vi "TestItemTo3Cam.vi"(0 "量测内容":string[][](array[string])) -> (3 "3只相机量测规格(不含取消的测试项目)":T4 {"相机4量测规格"."上限" format="%#.4g"; "相机4量测规格"."下限" format="%#.4g"; "相机3量测规格"."上限" format="%#.4g"; "相机3量测规格"."下限" format="%#.4g"; "相机2量测规格"."上限" format="%#.4g"; "相机2量测规格"."下限" format="%#.4g"; "相机1量测规格"."上限" format="%#.4g"; "相机1量测规格"."下限" format="%#.4g"}, 4 "各相机光源有效量测项目":T1, 6 "4只相机是否拍照":bool[](array[boolean]))   [LabVIEW 2014]
uses:
  CamLight.ctl
  Controls/TestThreshold.ctl
panel:
  out "数组 2":enum32{"相机1", "相机2", "相机3", "相机4"}[](array[ring])
  out "数组":bool[](array[boolean])
  out "第一次拍照组合":T2[](array[typedef])
  # "~"
  # "~"
  # "~"
  # "~"
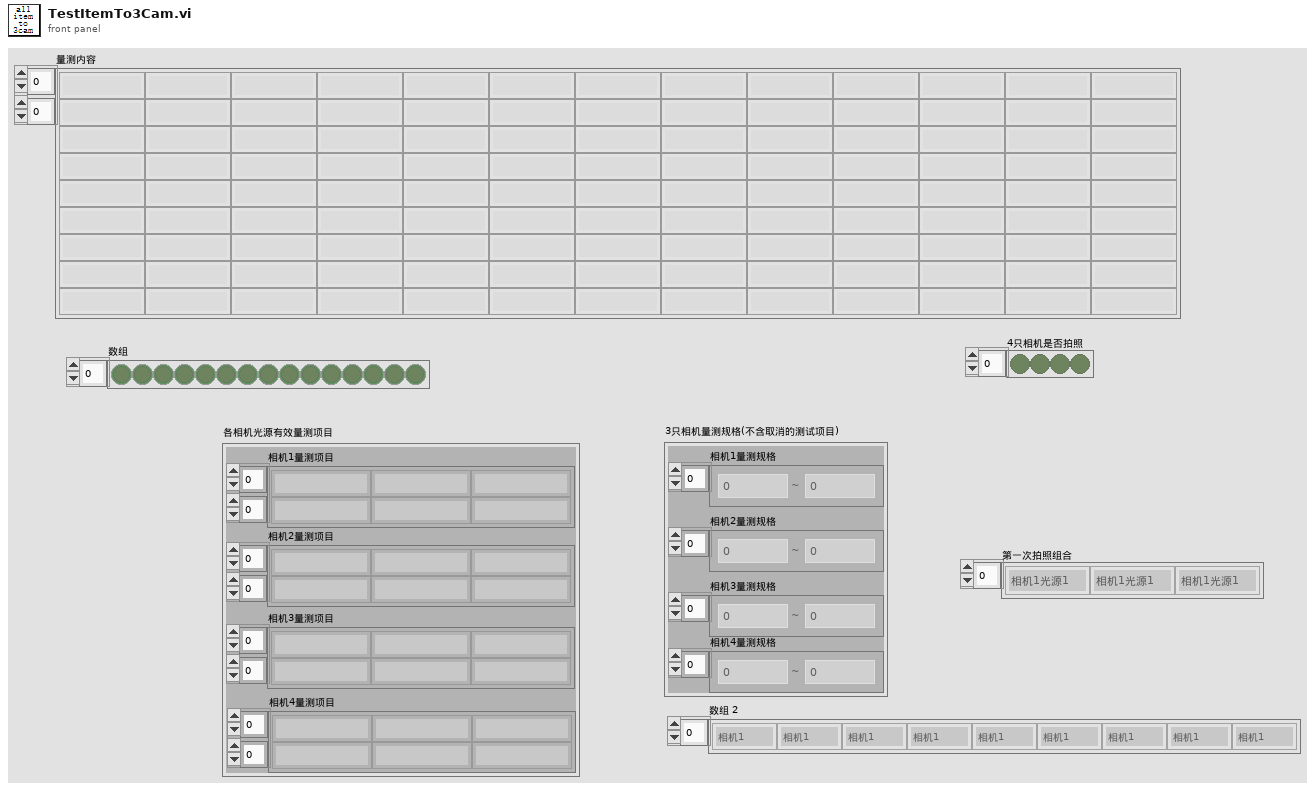
[diagram p1: front panel]
types:
  T1 = cluster{"相机1量测项目":string[][], "相机2量测项目":string[][], "相机3量测项目":string[][], "相机4量测项目":string[][]}
  T2 = typedef "CamLight.ctl" = enum16{"相机1光源1", "相机2光源2", "相机3光源3", "相机4光源4", "None"}
  T3 = typedef "TestThreshold.ctl" = cluster{"下限":dbl, "上限":dbl}
  T4 = cluster{"相机1量测规格":T3[], "相机2量测规格":T3[], "相机3量测规格":T3[], "相机4量测规格":T3[]}
  T5 = typedef "锁附点位信息.ctl" = cluster{"点位名称":string, "点位坐标(图纸)":T6, "点位坐标(实际)":T6, "补偿值":T6, "锁附时机械手角度":T7, "选择螺丝供料机":enum32{"1号供料机", "2号供料机", "3号供料机", "4号供料机"}}
  T6 = typedef "锁附点位坐标XYZ.ctl" = cluster{"X":dbl, "Y":dbl, "Z":dbl}
  T7 = typedef "锁附时机械手角度.ctl" = enum16{"0度", "90度", "180度", "270度"}
  T8 = cluster{string[][], string[][], string[][], string[][]}
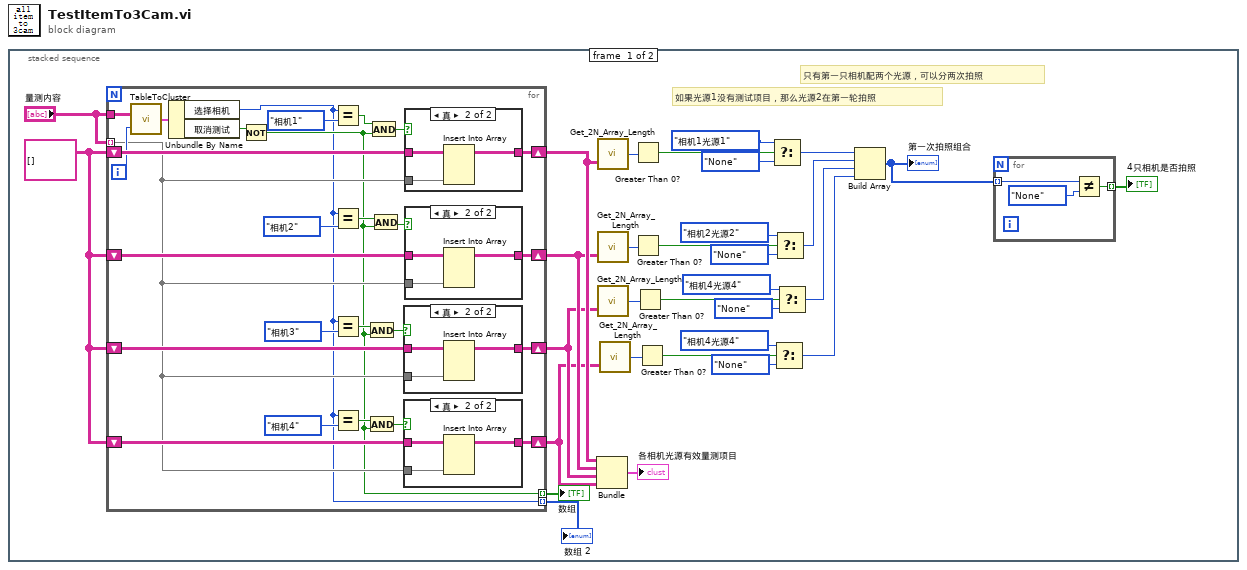
[diagram p0: block diagram]
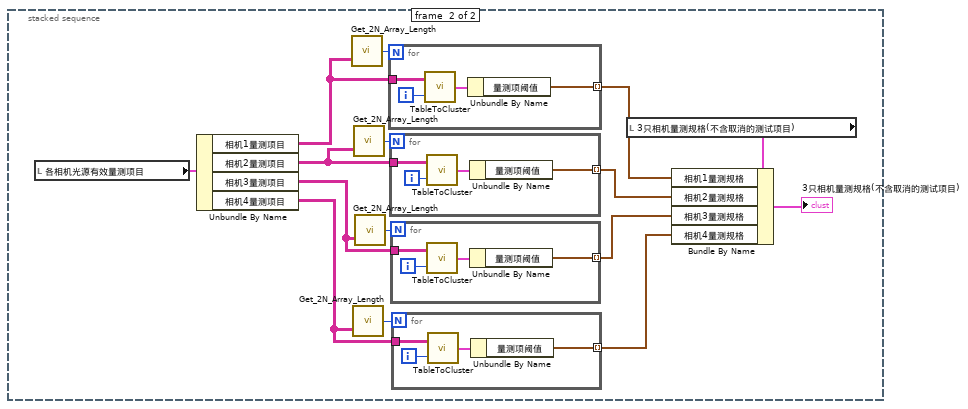
[diagram p6: hidden frame]
diagram:
  n1 = stacked-sequence {
    frame #0 {
      w12 = string[][] []
      # "只有第一只相机配两个光源，可以分两次拍照"
      # "如果光源1没有测试项目，那么光源2在第一轮拍照"
      n2 = for {
        tunnel: "量测内容" -> [w55]
        shift-right: [w60] -> w18
        shift-left: w12 -> [w61]
        shift-right: [w59] -> w17
        shift-left: w12 -> [w58]
        shift-right: [w57] -> w16
        shift-left: w12 -> [w56]
        tunnel: "量测内容" -> [w41] mode=indexing
        shift-right: [w42] -> w10
        shift-left: w12 -> [w43]
        tunnel: [w36] -> w2 mode=indexing
        tunnel: [w35] -> w1 mode=indexing
        i -> [w54]
        n3 = call "TableToCluster.vi"("Row"=w54, "锁附点位信息表"=w55) -> ("锁附点位信息"=w53:T5)
        n4 = Unbundle By Name(w53) -> ("选择相机"=w35:enum32{"相机1", "相机2", "相机3", "相机4"}, "取消测试"=w52:bool)
        n5 = Not(x=w52) -> (.not. x?=w36:bool)
        n6 = Equal?(x=w35, y=enum32{"相机1", "相机2", "相机3", "相机4"}."相机1") -> (x = y?=w51:bool)
        n7 = Equal?(x=w35, y=enum32{"相机1", "相机2", "相机3", "相机4"}."相机2") -> (x = y?=w49:bool)
        n8 = Equal?(x=w35, y=enum32{"相机1", "相机2", "相机3", "相机4"}."相机3") -> (x = y?=w47:bool)
        n9 = Equal?(x=w35, y=enum32{"相机1", "相机2", "相机3", "相机4"}."相机4") -> (x = y?=w44:bool)
        n10 = And(x=w47, y=w36) -> (x .and. y?=w46:bool)
        n11 = And(x=w44, y=w36) -> (x .and. y?=w45:bool)
        n12 = And(x=w51, y=w36) -> (x .and. y?=w50:bool)
        n13 = And(x=w49, y=w36) -> (x .and. y?=w48:bool)
        n14 = case shown="真" w46 {
          tunnel: w41 -> [_ w68]
          tunnel: w56 -> [w66 w69]
          tunnel: [w66 w67] -> w57
          frame False {
          }
          frame True {
            n15 = Insert Into Array(array=w69, new element=w68) -> (w67:string[][])  [unwired: 2 in]
          }
        }
        n16 = case shown="真" w45 {
          tunnel: w41 -> [_ w64]
          tunnel: w43 -> [w62 w65]
          tunnel: [w62 w63] -> w42
          frame False {
          }
          frame True {
            n17 = Insert Into Array(array=w65, new element=w64) -> (w63:string[][])  [unwired: 2 in]
          }
        }
        n18 = case shown="真" w50 {
          tunnel: w41 -> [_ w76]
          tunnel: w61 -> [w74 w77]
          tunnel: [w74 w75] -> w60
          frame False {
          }
          frame True {
            n19 = Insert Into Array(array=w77, new element=w76) -> (w75:string[][])  [unwired: 2 in]
          }
        }
        n20 = case shown="真" w48 {
          tunnel: w41 -> [_ w72]
          tunnel: w58 -> [w70 w73]
          tunnel: [w70 w71] -> w59
          frame False {
          }
          frame True {
            n21 = Insert Into Array(array=w73, new element=w72) -> (w71:string[][])  [unwired: 2 in]
          }
        }
      }
      "数组" <- w2
      "数组 2" <- w1
      n22 = Bundle(w18, w17, w16, w10) -> (→"各相机光源有效量测项目":T8)  [unwired: 1 in]
      n23 = call "Get_2N_Array_Length.vi"("StringArray"=w18) -> ("Numeric"=w31:i32)  [unwired: 1 in]
      n24 = call "Get_2N_Array_Length.vi"("StringArray"=w17) -> ("Numeric"=w30:i32)  [unwired: 1 in]
      n25 = call "Get_2N_Array_Length.vi"("StringArray"=w16) -> ("Numeric"=w29:i32)  [unwired: 1 in]
      n26 = call "Get_2N_Array_Length.vi"("StringArray"=w10) -> ("Numeric"=w11:i32)  [unwired: 1 in]
      n27 = Greater Than 0?(x=w31) -> (x > 0?=w25:bool)
      n28 = Greater Than 0?(x=w30) -> (x > 0?=w24:bool)
      n29 = Greater Than 0?(x=w29) -> (x > 0?=w23:bool)
      n30 = Greater Than 0?(x=w11) -> (x > 0?=w6:bool)
      n31 = Select(t=CamLight."相机1光源1", s=w25, f=CamLight."None") -> (s? t:f=w22:T2)
      n32 = Select(t=CamLight."相机4光源4", s=w6, f=CamLight."None") -> (s? t:f=w5:T2)
      n33 = Select(t=CamLight."相机2光源2", s=w24, f=CamLight."None") -> (s? t:f=w21:T2)
      n34 = Select(t=CamLight."相机4光源4", s=w23, f=CamLight."None") -> (s? t:f=w20:T2)
      n35 = Build Array(w22, w21, w20, w5) -> (w19:T2[])
      "第一次拍照组合" <- w19
      n36 = for {
        tunnel: w19 -> [w34] mode=indexing
        tunnel: [w32] -> w4 mode=indexing
        n37 = Not Equal?(x=w34, y=CamLight."None") -> (x != y?=w32:bool)
      }
      "4只相机是否拍照" <- w4
    }
    frame #1 {
      n38 = local read "各相机光源有效量测项目"() -> (w86:T1)
      n39 = Unbundle By Name(w86) -> ("相机1量测项目"=w85:string[][], "相机2量测项目"=w83:string[][], "相机3量测项目"=w80:string[][], "相机4量测项目"=w79:string[][])
      n40 = call "Get_2N_Array_Length.vi"("StringArray"=w85) -> ("Numeric"=w84:i32)  [unwired: 1 in]
      n41 = call "Get_2N_Array_Length.vi"("StringArray"=w79) -> ("Numeric"=w78:i32)  [unwired: 1 in]
      n42 = call "Get_2N_Array_Length.vi"("StringArray"=w83) -> ("Numeric"=w82:i32)  [unwired: 1 in]
      n43 = call "Get_2N_Array_Length.vi"("StringArray"=w80) -> ("Numeric"=w81:i32)  [unwired: 1 in]
      n44 = for {
        N: w84 -> [_]
        tunnel: [w105] -> w90 mode=indexing
        tunnel: w85 -> [w108]
        i -> [w107]
        n45 = call "TableToCluster.vi"("Row"=w107, "锁附点位信息表"=w108) -> ("锁附点位信息"=w106:T5)
        n46 = Unbundle By Name(w106) -> ("量测项阈值"=w105:T3)
      }
      n47 = for {
        N: w82 -> [_]
        tunnel: w83 -> [w103]
        tunnel: [w101] -> w91 mode=indexing
        i -> [w102]
        n48 = call "TableToCluster.vi"("Row"=w102, "锁附点位信息表"=w103) -> ("锁附点位信息"=w104:T5)
        n49 = Unbundle By Name(w104) -> ("量测项阈值"=w101:T3)
      }
      n50 = for {
        N: w81 -> [_]
        tunnel: w80 -> [w99]
        tunnel: [w97] -> w92 mode=indexing
        i -> [w98]
        n51 = call "TableToCluster.vi"("Row"=w98, "锁附点位信息表"=w99) -> ("锁附点位信息"=w100:T5)
        n52 = Unbundle By Name(w100) -> ("量测项阈值"=w97:T3)
      }
      n53 = for {
        N: w78 -> [_]
        tunnel: w79 -> [w95]
        tunnel: [w93] -> w87 mode=indexing
        i -> [w94]
        n54 = call "TableToCluster.vi"("Row"=w94, "锁附点位信息表"=w95) -> ("锁附点位信息"=w96:T5)
        n55 = Unbundle By Name(w96) -> ("量测项阈值"=w93:T3)
      }
      n56 = local read "3只相机量测规格(不含取消的测试项目)"() -> (w88:T4)
      n57 = Bundle By Name(cluster=w88, "相机1量测规格"=w90, "相机2量测规格"=w91, "相机3量测规格"=w92, "相机4量测规格"=w87) -> (→"3只相机量测规格(不含取消的测试项目)":T4)
    }
  }
